vi "Vision Research Phantom Series PhCon PhSendTrigger.vi"(0 "CN in":u32=1, 5 "Error In (no error)":errorcluster) -> (14 "CN out":u32=1, 19 "Error Out":errorcluster)   [LabVIEW 2013, in "VRI.lvlib"]
doc: "PhCon dll\n\nPhSendTrigger\nHRESULT PhSendTrigger(UINT CN);\n\nParameters Description\nCN (in) Camera number.\nReturn HRESULT (0=Ok)\nComments Send a software trigger to the camera. \n This is a handy way to finish a recording.\n\nWritten by:\nBLOOMY CONTROLS, INC\nWINDSOR, CT 06095, USA\n860-298-9925\nwww.bloomy.com\nV1.0.0\nMay, 2004"
uses:
  VRI.lvlib
  Phantom DLLs/PhCon.Dll
panel:
  # "For instructions on the use of this VI, press Ctrl+H to display the help window and move the mouse over the icon, controls, and indicators"
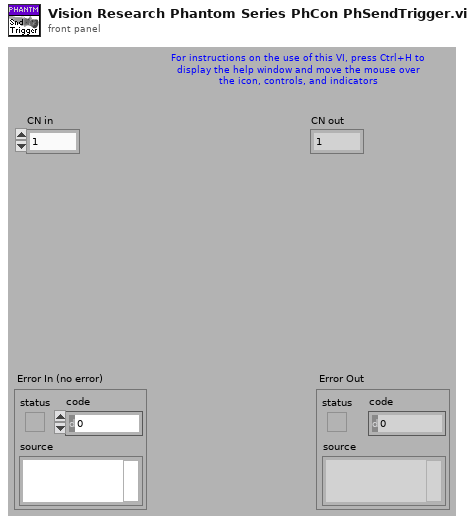
[diagram p1: front panel]
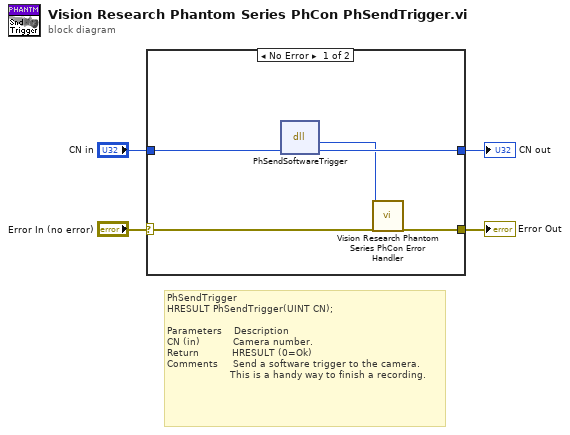
[diagram p0: block diagram]
diagram:
  # "PhSendTrigger\nHRESULT PhSendTrigger(UINT CN);\n\nParameters    Description\nCN (in)           Camera number.\nReturn           HRESULT (0=Ok)\nComments     Send a software trigger to the camera. \n                     This is a handy way to finish a recording."
  n1 = case shown="No Error" "Error In (no error)" {
    selector: "Error In (no error)" -> [w9 w11]
    tunnel: [w8 w11] -> w3
    tunnel: "CN in" -> [w7 w10]
    tunnel: [w6 w10] -> w1
    frame No Error {
      n2 = dll-call lib="C:/Projects/SDK/64-bit/Vision Research Phantom Series Labview Driver/Phantom DLLs/PhCon.dll" fn="PhSendSoftwareTrigger"("CN"=w7) -> ("HRESULT"=w5:i32, "CN"=w6:u32)  [unwired: 3 in, 2 out]
      n3 = call "Vision Research Phantom Series PhCon Error Handler.vi"("ErrNo"=w5, "Error In (no error)"=w9) -> ("Error Out"=w8:errorcluster)  [unwired: 17 out]
    }
    frame Error {
    }
  }
  "Error Out" <- w3
  "CN out" <- w1
